vi "Device Launcher.vi"(0 "Notifier Name":string="Not a Name", 7 "Device Ports/IDs/Channels":string[](array[string]), 11 "Device Engine Path":path) -> (4 "Notifier Name":string, 15 "Running?":bool)   [LabVIEW 2016]
uses:
  Device Launcher Controls/Device Information.ctl
panel:
  out "Error?":bool
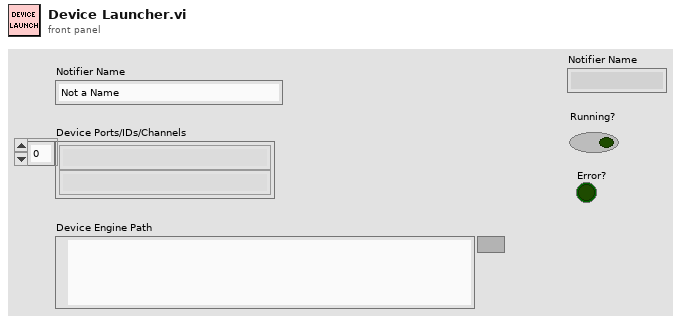
[diagram p1: front panel]
types:
  T1 = typedef "Device Information.ctl" = cluster{"Notifier Name":string, "Device Ports/IDs/Channels":string[], "Device Engine Path":path}
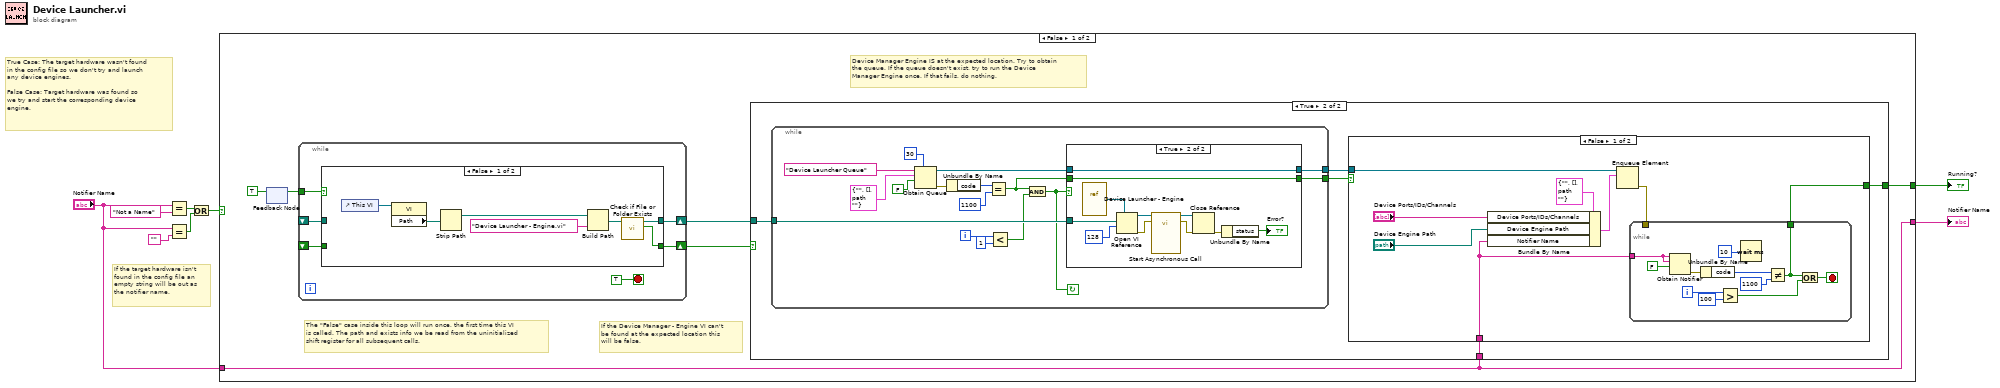
[diagram p0: block diagram]
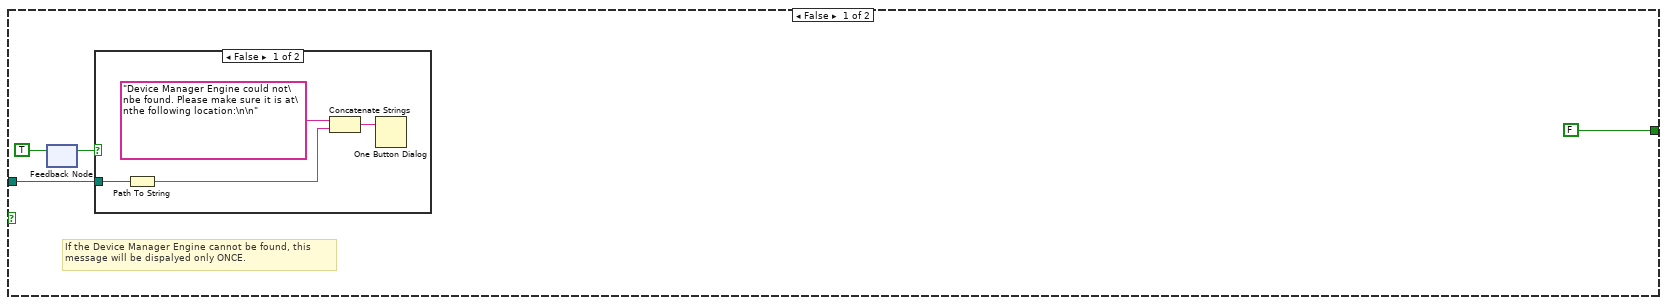
[diagram p2: hidden frame]
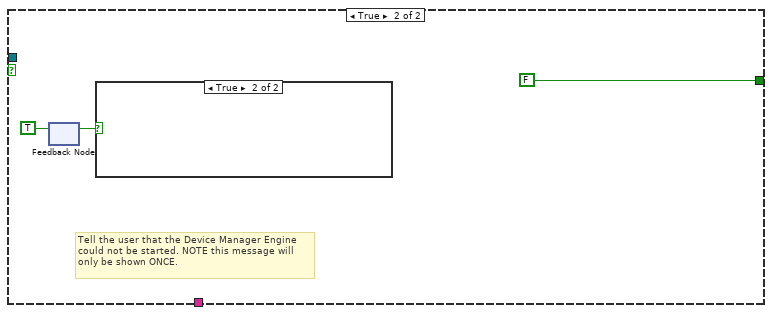
[diagram p4: hidden frame]
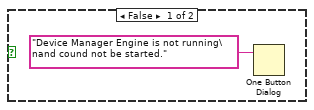
[diagram p5: hidden frame]
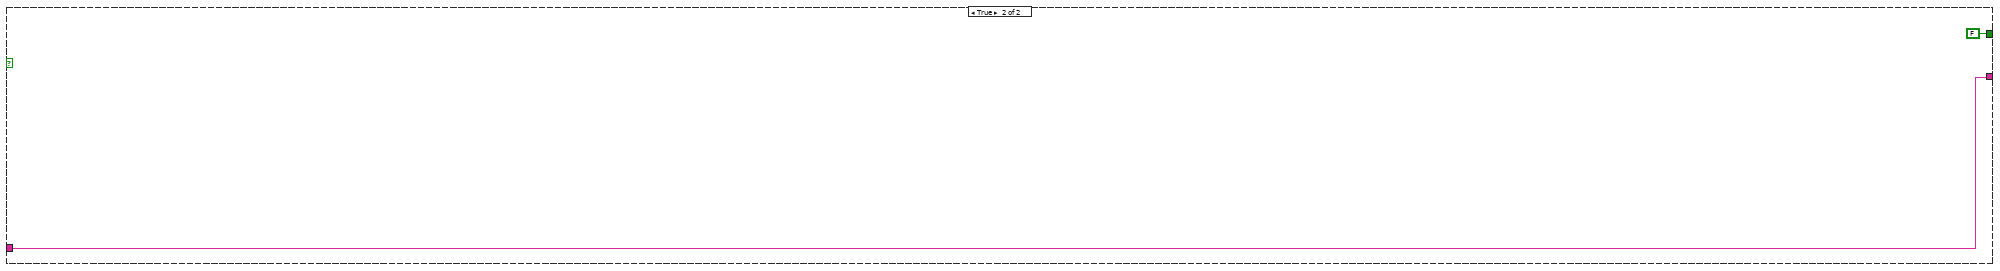
[diagram p8: hidden frame]
diagram:
  # "True Case: The target hardware wasn't found\nin the config file so we don't try and launch\nany device engines.\n\nFalse Case: Target hardware was found so\nwe try and start the corresponding device\nengine."
  # "If the target hardware isn't\nfound in the config file an\nempty string will be out as\nthe notifier name."
  n1 = Equal?(x="Notifier Name", y="Not a Name") -> (x = y?=w6:bool)
  n2 = Equal?(x="Notifier Name", y="") -> (x = y?=w5:bool)
  n3 = Or(x=w6, y=w5) -> (x .or. y?=w4:bool)
  n4 = case shown="False" w4 {
    tunnel: [w10 FALSE] -> w8
    tunnel: "Notifier Name" -> [w9 w96]
    tunnel: [w9 w96] -> w1
    frame False {
      # "Device Manager Engine IS at the expected location. Try to obtain\nthe queue. If the queue doesn't exist, try to run the Device\nManager Engine once. If that fails, do nothing."
      # "If the Device Manager - Engine VI can't\nbe found at the expected location this\nwill be false."
      # "The \"False\" case inside this loop will run once, the first time this VI\nis called. The path and exists info we be read from the uninitialized\nshift register for all subsequent calls."
      n5 = feedback #1() -> (w14:bool)  [unwired: 1 in]
      n6 = feedback-in #1(TRUE) -> ()
      n7 = while {
        shift-right: [w84] -> w12
        shift-left: _ -> [w82]
        shift-right: [w83] -> w11
        shift-left: _ -> [w81]
        tunnel: w14 -> [w80]
        stop <- TRUE stop-if-true
        n8 = case shown="False" w80 {
          tunnel: [w87 w94] -> w84
          tunnel: [w86 w93] -> w83
          tunnel: w82 -> [_ w94]
          tunnel: w81 -> [_ w93]
          frame False {
            n9 = control-ref of="This VI"() -> (w92:refnum<vi>)
            n10 = property class="VI"(reference=w92) -> ("Path"=w91:path)  [unwired: 1 in, 2 out]
            n11 = Strip Path(path=w91) -> (stripped path=w90:path)  [unwired: 1 out]
            n12 = Build Path(base path=w90, name or relative path="Device Launcher - Engine.vi" ("name (unnamed)")) -> (appended path=w88:path)
            n13 = call <vilib>:"Check if File or Folder Exists.vi"("path"=w88) -> ("file or folder exists?"=w86:bool, "dup path"=w87:path)  [unwired: 8 in, 1 out]
          }
          frame True {
          }
        }
      }
      n14 = case shown="True" w11 {
        tunnel: w12 -> [w16 w27]
        tunnel: [FALSE w24] -> w10
        tunnel: w9 -> [_ w23]
        frame False {
          # "If the Device Manager Engine cannot be found, this\nmessage will be dispalyed only ONCE."
          n15 = feedback-in #2(TRUE) -> ()
          n16 = feedback #2() -> (w17:bool)  [unwired: 1 in]
          n17 = case shown="False" w17 {
            tunnel: w16 -> [w21 _]
            frame False {
              n18 = Path To String(path=w21) -> (string=w20:string)
              n19 = Concatenate Strings("Device Manager Engine could not\nbe found. Please make sure it is at\nthe following location:\n\n", w20) -> (w19:string)
              n20 = One Button Dialog(message=w19) -> ()  [unwired: 1 in, 1 out]
            }
            frame True {
            }
          }
        }
        frame True {
          n21 = while {
            tunnel: w27 -> [w59]
            tunnel: [w56] -> w26
            tunnel: [w55] -> w25
            i -> [w58]
            stop <- w51 continue-if-true
            n22 = Obtain Queue(max queue size (-1, unlimited)=30, name (unnamed)="Device Launcher Queue", element data type=T1 {"Notifier Name"="", "Device Ports/IDs/Channels"=[], "Device Engine Path"=path ""} ("Device Information"), create if not found? (T)=FALSE) -> (queue out=w66:refnum<queue>, error out=w64:errorcluster)  [unwired: 1 in, 1 out]
            n23 = Unbundle By Name(w64) -> ("code"=w65:i32)
            n24 = Equal?(x=w65, y=1100) -> (x = y?=w52:bool)
            n25 = Less?(x=w58, y=1) -> (x < y?=w53:bool)
            n26 = And(x=w52, y=w53) -> (x .and. y?=w51:bool)
            n27 = case shown="True" w51 {
              tunnel: w66 -> [w68 w78]
              tunnel: w59 -> [_ w79]
              tunnel: [w68 w78] -> w55
              tunnel: w52 -> [w67 w77]
              tunnel: [w67 w77] -> w56
              frame False {
              }
              frame True {
                n28 = vi-ref "Device Launcher - Engine.vi"() -> (w73:refnum<vi>)
                n29 = Open VI Reference(type specifier VI Refnum (for type only)=w73, vi path=w79, options=128) -> (vi reference=w72:refnum<vi>, error out=w70:errorcluster)  [unwired: 3 in]
                n30 = call-by-ref "Start Asynchronous Call"(reference=w72, error in=w70) -> (reference out=w71:refnum<vi>, error out=w69:errorcluster)  [unwired: 12 in]
                n31 = Close Reference(reference=w71, error in (no error)=w69) -> (error out=w76:errorcluster)
                n32 = Unbundle By Name(w76) -> ("status"=→"Error?":bool)
              }
            }
          }
          n33 = case shown="False" w26 {
            tunnel: w25 -> [w32 _]
            tunnel: [w30 FALSE] -> w24
            tunnel: w23 -> [w28 _]
            frame False {
              n34 = Bundle By Name(cluster=T1 {"Notifier Name"="", "Device Ports/IDs/Channels"=[], "Device Engine Path"=path ""} ("Device Information"), "Device Ports/IDs/Channels"="Device Ports/IDs/Channels", "Device Engine Path"="Device Engine Path", "Notifier Name"=w28) -> (w31:T1)
              n35 = Enqueue Element(queue=w32, element=w31) -> (error out=w29:errorcluster)  [unwired: 2 in, 2 out]
              n36 = while {
                tunnel: w28 -> [w46]
                tunnel: [w36] -> w30
                tunnel: w29 -> [_]
                i -> [w42]
                stop <- w37 stop-if-true
                n37 = Obtain Notifier(name (unnamed)=w46, notification data type=w46, create if not found? (T)=FALSE) -> (error out=w44:errorcluster)  [unwired: 1 in, 2 out]
                n38 = Unbundle By Name(w44) -> ("code"=w41:i32)
                n39 = Greater?(x=w42, y=100) -> (0:w38:bool)
                n40 = Wait (ms)(milliseconds to wait=u32 10) -> ()  [unwired: 1 out]
                n41 = Not Equal?(x=w41, y=1100) -> (x != y?=w36:bool)
                n42 = Or(x=w36, y=w38) -> (x .or. y?=w37:bool)
              }
            }
            frame True {
              # "Tell the user that the Device Manager Engine\ncould not be started. NOTE this message will\nonly be shown ONCE."
              n43 = feedback #3() -> (w47:bool)  [unwired: 1 in]
              n44 = feedback-in #3(TRUE) -> ()
              n45 = case shown="True" w47 {
                frame False {
                  n46 = One Button Dialog(message="Device Manager Engine is not running\nand cound not be started.") -> ()  [unwired: 1 in, 1 out]
                }
                frame True {
                }
              }
            }
          }
        }
      }
    }
    frame True {
    }
  }
  "Running?" <- w8
  "Notifier Name" <- w1
